vi "extension-remover.vi"(10 "path":path) -> (2 "w/o extension":string="^(.+)\\.[a-z0-9]+$")   [LabVIEW 2017]
uses:
  <vilib>/regexp/Match Regular Expression.xnode
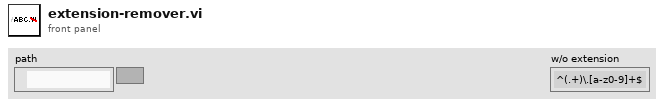
[diagram p1: front panel]
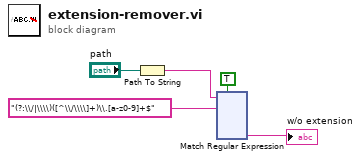
[diagram p0: block diagram]
diagram:
  n1 = Path To String(path="path") -> (string=w2:string)
  n2 = xnode "Match Regular Expression"("input string"=w2, "regular expression"="(?:\\/|\\\\)([^\\/\\\\]+)\\.[a-z0-9]+$", "ignore case? (F)"=TRUE) -> ("submatch 1"=→"w/o extension":string)  [unwired: 3 in, 5 out]
